vi "Create and Save Signal.vi"   [LabVIEW 2015]
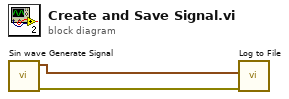
[diagram p0: block diagram]
diagram:
  n1 = call "Sin wave Generate Signal.vi"() -> ("error out"=w1:errorcluster, "Waveform Graph"=w2:waveform(dbl))  [unwired: 10 in]
  n2 = call "Log to File.vi"("error in"=w1, "Waveform Graph"=w2) -> ()  [unwired: 9 in, 1 out]
